vi "test_CCDParseChipSize.vi"() -> ()   [LabVIEW 2023]
uses:
  Classes/CCD/Chipsize.ctl
  74a40d5a-e2eb-476d-a2c2-0a4e45cf5566.vi
  <vilib>/JDP Science/JSONtext/JSON text to Variant.vi
  <vilib>/addons/_JKI Toolkits/Caraya/classes/Assert/Assert Equal Value_Variant.vi
  <vilib>/addons/_JKI Toolkits/Caraya/classes/Assert/Assert Not Error.vi
  <vilib>/JDP Science/JSONtext/LVClass Serializer/JSONtext LVClass Serializer.lvclass
  Classes/CCD/CCD.lvclass
  Classes/Communicator/Communicator.lvclass
  <vilib>/addons/_JKI Toolkits/Caraya/classes/Test/Test.lvclass
  <vilib>/addons/_JKI Toolkits/Caraya/classes/Assert/Assert.lvclass
panel:
  out "error out":errorcluster
  out "<JSON>":string caption="JSON.result"
  out "Data out":T1
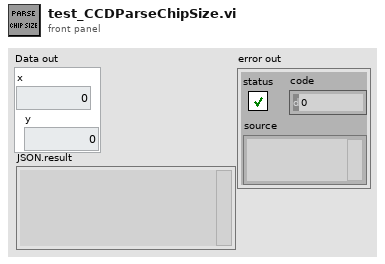
[diagram p1: front panel]
types:
  T1 = typedef "CCD.lvclass/Chipsize.ctl" = cluster{"x":i32, "y":i32}
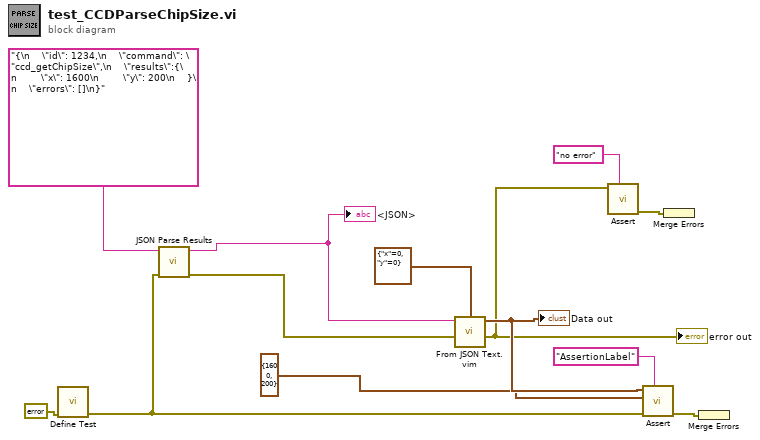
[diagram p0: block diagram]
diagram:
  n1 = call <vilib>:"Define Test.vi"("error in (no error)"=errorcluster {"status"=FALSE, "code"=0, "source"=""}) -> ("error out"=w7:errorcluster)  [unwired: 9 in, 1 out]
  n2 = call "JSON Parse Results.vi"("error in (no error)"=w7, "JSON"="{\n    \"id\": 1234,\n    \"command\": \"ccd_getChipSize\",\n    \"results\":{\n        \"x\": 1600\n        \"y\": 200\n    }\n    \"errors\": []\n}") -> ("error out"=w12:errorcluster, "results-JSON"=w4:string)  [unwired: 7 in, 1 out]
  "<JSON>" <- w4
  n3 = call "From JSON Text.vim"("Data Type and Default Value"=T1 {"x"=0, "y"=0} ("Chipsize"), "error in (no error)"=w12, "JSON"=w4) -> ("error out"=w1:errorcluster, "Data out"=w6:T1)  [unwired: 7 in]
  "Data out" <- w6
  "error out" <- w1
  n4 = call-poly <vilib>:"Assert.vi"("Label"="no error" ("Label (VI Title)"), "Not Error?"=w1) -> ("error out"=w2:errorcluster)  [unwired: 8 in, 1 out]
  n5 = call-poly <vilib>:"Assert.vi"("Label"="AssertionLabel" ("Label (VI Title)"), "error in (no error)"=w7, "Y"=T1 {"x"=1600, "y"=200} ("Data out"), "X"=w6) -> ("error out"=w10:errorcluster)  [unwired: 6 in, 1 out]
  n6 = Merge Errors(w2) -> ()  [unwired: 1 out]
  n7 = Merge Errors(w10) -> ()  [unwired: 1 out]
